vi "Filter Multi DLL (SubVI).vi"(8 "error in (no error)":errorcluster, 11 "Robot State Charts In":path[](array[path])) -> (0 "error out":errorcluster, 3 "Robot State Charts Out":path[](array[path]))   [LabVIEW 2014]
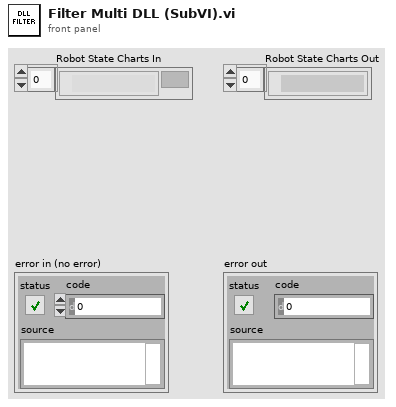
[diagram p1: front panel]
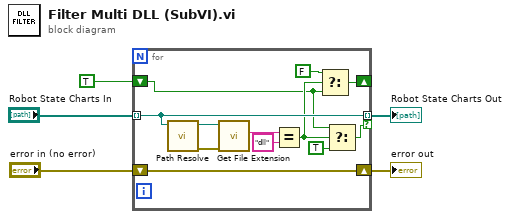
[diagram p0: block diagram]
diagram:
  n1 = for {
    tunnel: "Robot State Charts In" -> [w14] mode=indexing
    tunnel: [w14] -> w3 mode=indexing if=w11
    shift-right: [w17] -> w5
    shift-left: "error in (no error)" -> [w17]
    shift-right: [w9] -> _
    shift-left: TRUE -> [w6]
    n2 = call "Path Resolve.vi"("absolute or relative path"=w14) -> ("Error Out"=w15:errorcluster, "resolved path"=w16:path)  [unwired: 9 in]
    n3 = call <vilib>:"Get File Extension.vi"("error in (no error)"=w15, "file"=w16) -> ("lowercase file extension"=w13:string)  [unwired: 6 in, 3 out]
    n4 = Equal?(x=w13, y="dll") -> (x = y?=w8:bool)
    n5 = Select(t=FALSE, s=w8, f=w6) -> (s? t:f=w9:bool)
    n6 = Select(t=w6, s=w8, f=TRUE) -> (s? t:f=w11:bool)
  }
  "error out" <- w5
  "Robot State Charts Out" <- w3
